vi "Stats.vi"() -> (0 "Collisions":i32[](array[numeric]), 1 "Kills":i32[](array[numeric]), 2 "Generated":i32[](array[numeric]), 3 "Squares":i32[](array[numeric]), 4 "Players":string[](array[string]))   [LabVIEW 2015, in "Square.lvclass"]
uses:
  Square.lvclass
  SubVIs/SB SubVIs.lvlib
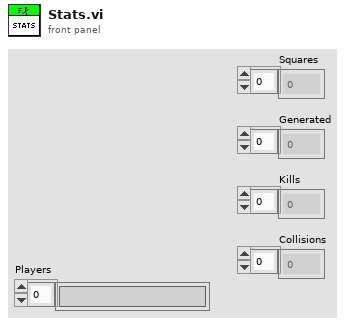
[diagram p1: front panel]
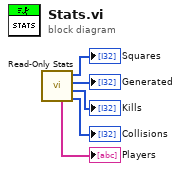
[diagram p0: block diagram]
diagram:
  n1 = call "Read-Only Stats.vi"() -> ("Collisions"=→"Collisions":i32[], "Kills"=→"Kills":i32[], "Generated"=→"Generated":i32[], "Squares"=→"Squares":i32[], "Players"=→"Players":string[])  [unwired: 7 in]
